vi "Read FPGA DIO.vi"(8 "error in":errorcluster, 11 "FPGA-DIO in":refnum<class "FPGA_DIO.lvclass">) -> (0 "error out":errorcluster, 1 "Port Array":u8[](array[numeric]), 2 "Boolean array":bool[](array[boolean]), 3 "FPGA-DIO out":refnum<class "FPGA_DIO.lvclass">)   [LabVIEW 2019, in "FPGA_DIO.lvlib" / "FPGA_DIO.lvclass"]
uses:
  Library/FPGA_DIO.lvclass
  C:/Users/Public/Documents/Development/builds/Instruments/DIG_IO.lvlibp/Library/DIG_IO.lvclass
  Library/FPGA_DIO.lvclass/FPGA_DIO.ctl
  builds/Instruments/DIG_IO.lvlibp/Accessors/Read Banks.vi
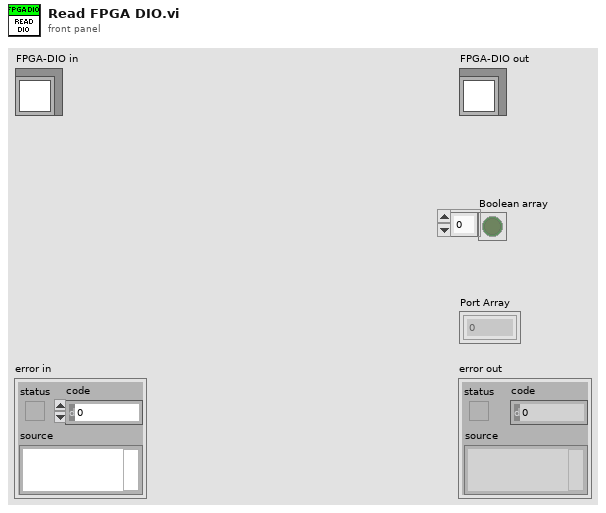
[diagram p1: front panel]
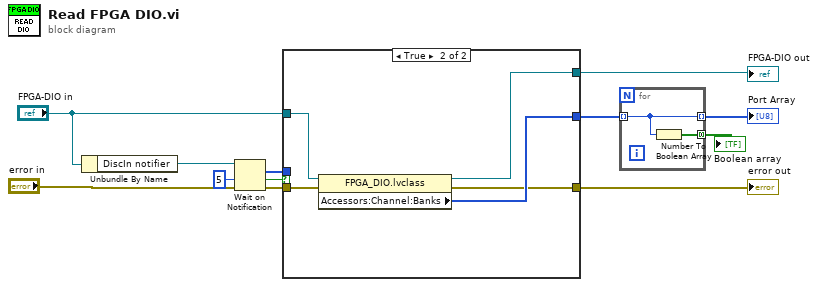
[diagram p0: block diagram]
diagram:
  n1 = Unbundle By Name("FPGA-DIO in") -> ("DiscIn notifier"=w12:refnum<notifier>)
  n2 = Wait on Notification(notifier=w12, timeout in ms (-1)=5, error in (no error)="error in") -> (notification=w8:u8[], timed out?=w9:bool, error out=w7:errorcluster)  [unwired: 1 in, 1 out]
  n3 = case shown="True" w9 {
    tunnel: w8 -> [w13 _]
    tunnel: w7 -> [w15 w17]
    tunnel: "FPGA-DIO in" -> [w14 w20]
    tunnel: [w14 w19] -> w5
    tunnel: [w13 w18] -> w3
    tunnel: [w15 w16] -> w4
    frame False {
    }
    frame True {
      n4 = property class="FPGA_DIO.lvclass"(reference=w20, error in=w17) -> (reference out=w19:refnum<class "FPGA_DIO.lvclass">, error out=w16:errorcluster, "Accessors:Channel:Banks"=w18:u8[])
    }
  }
  "error out" <- w4
  "FPGA-DIO out" <- w5
  n5 = for {
    tunnel: w3 -> [w22] mode=indexing
    tunnel: [w22] -> w2 mode=indexing
    tunnel: [w21] -> w1 mode=concatenating
    n6 = Number To Boolean Array(number=w22) -> (Boolean array=w21:bool[])
  }
  "Port Array" <- w2
  "Boolean array" <- w1
